vi "delete_Instrument.FrameworkTemplate.AppLauncher.vi"(8 "error in":errorcluster, 10 "Configuration Window? [T]":bool=TRUE, 11 "Debug Mode? [F]":bool) -> (0 "error out":errorcluster)   [LabVIEW 2019]
uses:
  <vilib>/JKI/JKI SMO/SMO/Typedefs/SMOState --Enum.ctl
  <userlib>/LevyLab/Instrument Framework/SMOs/Instrument/Instrument.lvclass
  C:/Program Files (x86)/National Instruments/LabVIEW 2019/vi.lib/JKI/JKI SMO/SMO/SMO.lvclass
  <userlib>/LevyLab/Instrument Framework/SMOs/Instrument UI/Instrument UI.lvclass
  C:/Program Files (x86)/National Instruments/LabVIEW 2019/vi.lib/JKI/JKI SMO/SMO.UI/SMO.UI.lvclass
  Instrument UI.FrameworkTemplate/Instrument UI.FrameworkTemplate.lvclass
  C:/Program Files (x86)/National Instruments/LabVIEW 2019/user.lib/LevyLab/Instrument Framework/SMOs/Instrument UI/Instrument UI.lvclass
  Instrument.FrameworkTemplate.lvclass
  C:/Program Files (x86)/National Instruments/LabVIEW 2019/user.lib/LevyLab/Instrument Framework/SMOs/Instrument/Instrument.lvclass
  <vilib>/JKI/JKI SMO/SMO/SMO.lvclass/SMO.ctl
  <vilib>/JKI/JKI SMO/SMO/Private/ReftoDVR--SMO.vi
  <vilib>/JKI/JKI SMO/SMO/SMO.lvclass
  <vilib>/JKI/JKI SMO/SMO.UI/SMO.UI.lvclass
panel:
  in  "Splash Status":string="Push Start to Start..." caption="String"
  in  "Start":bool=TRUE
  in  "Stop":bool=TRUE
  out "UI SMO State":T1=enum."Stopped"
  out "SMO State":T1
  # "Example Instrument SMO Test Launcher"
  # "For instructions on how to use the JKI State Machine Objects, examples and video tutorials, visit:\nhttp://jki.net/state-machine-objects/\n\nJKI State Machine Objects™\nhttp://jki.net/state-machine-objects/\nCopyright (C) 2005-2015, JKI <info@jki.net>\nALL RIGHTS RESERVED"
  # "Starting Example Instrument..."
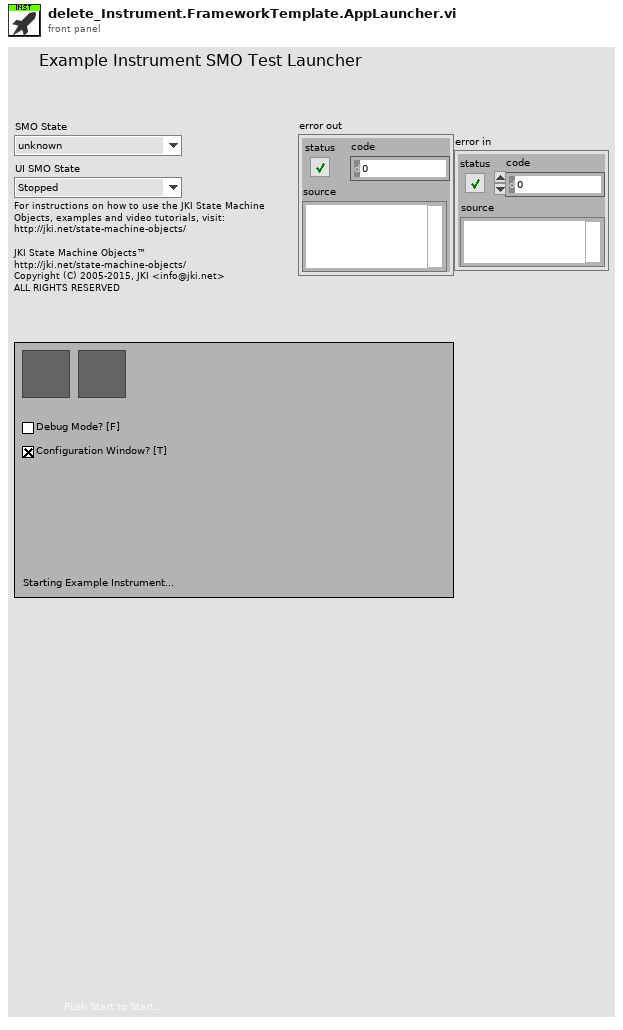
[diagram p1: front panel]
types:
  T1 = typedef "SMO.lvclass/SMOState --Enum.ctl" = enum16{"unknown", "Created", "Started", "Stopped"}
  T2 = enum32{"Invalid", "Standard", "Closed", "Hidden", "Minimized", "Maximized"}
  T3 = enum32{"invalid app kind", "Development System", "Run Time System", "Student Edition", "Embedded LabVIEW", "Evaluation", "Custom"}
  T4 = cluster{"Core":cluster{"Current VI Reference":refnum<vi>, "Close Panel on Exit?":bool}, "Instrument":refnum<class "Instrument.lvclass">, "Instrument UI":refnum<class "Instrument UI.lvclass">}
  T5 = cluster{"Current VI Reference":refnum<vi>, "Close Panel on Exit?":bool}
  T6 = typedef "SMO.lvclass/Public Events.ctl" = cluster{"Error":refnum<user-event>, "State":refnum<user-event>, "Reserve State":refnum<user-event>}
  T7 = cluster{"Event Registration Refnum":refnum<event-registration>, "Event Registration Refnum":refnum<event-registration>}
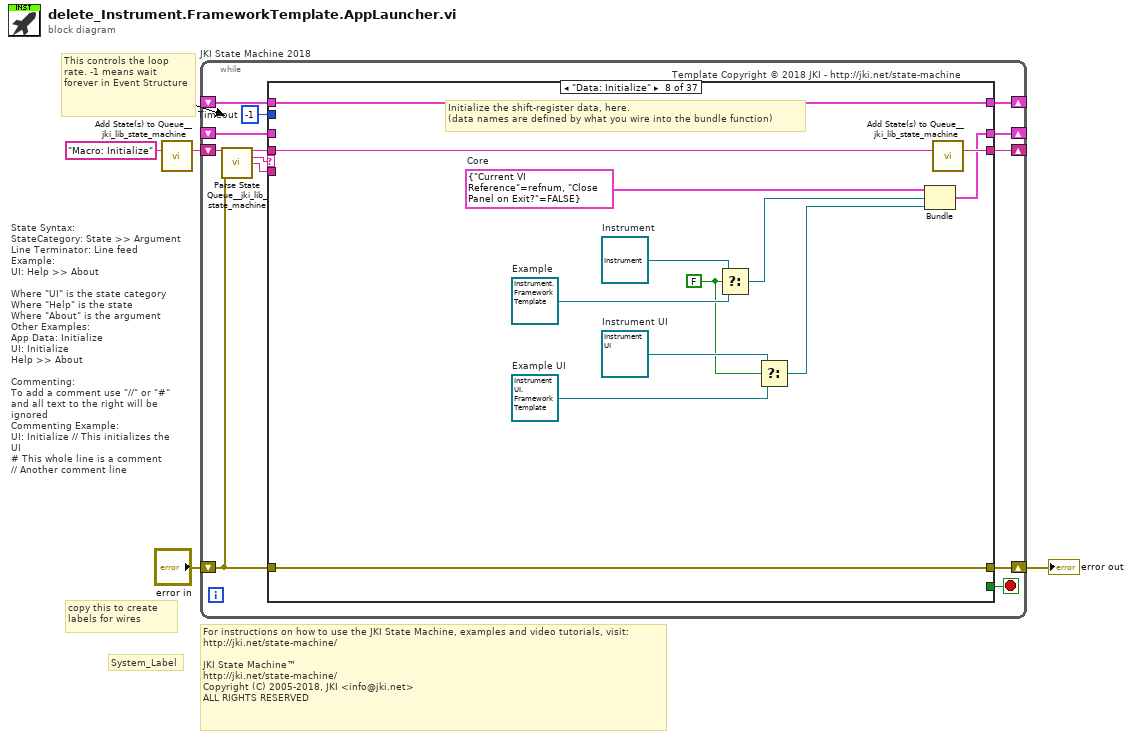
[diagram p0: block diagram]
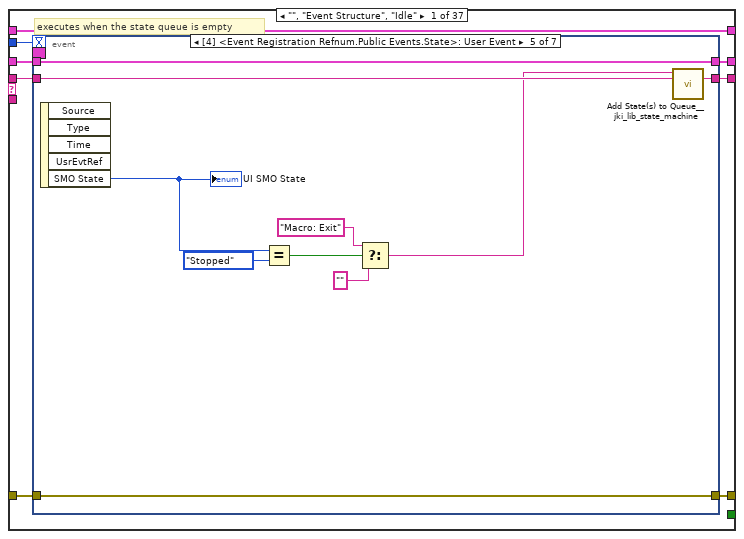
[diagram p2: hidden frame]
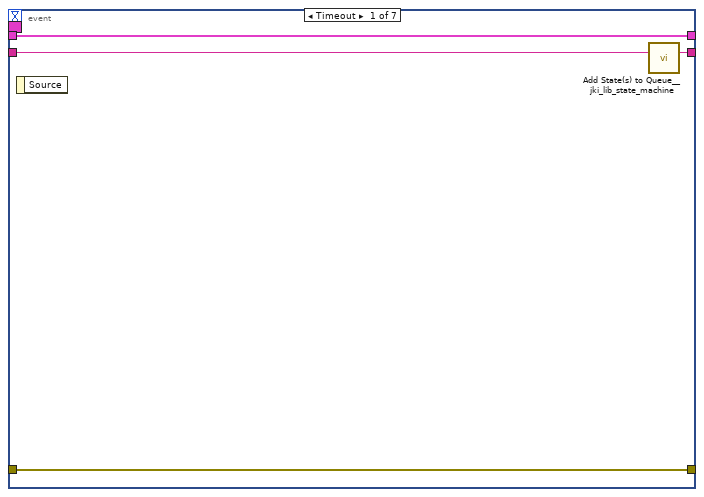
[diagram p3: hidden frame]
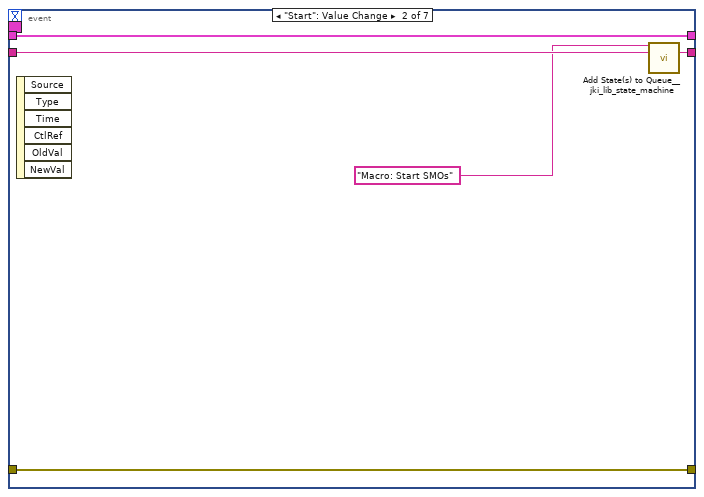
[diagram p4: hidden frame]
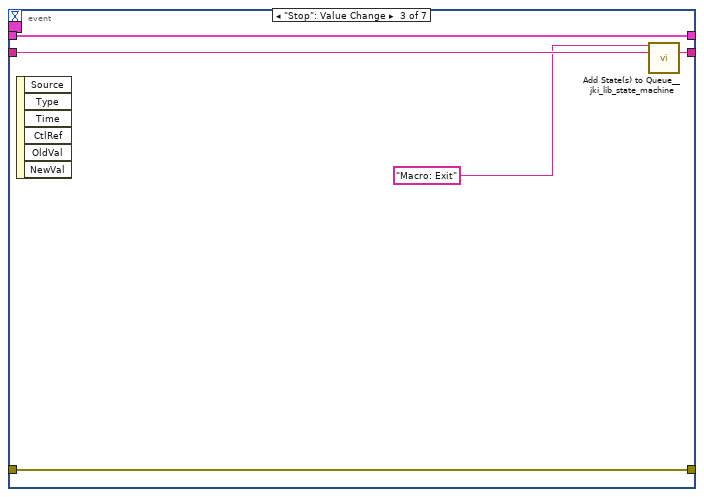
[diagram p5: hidden frame]
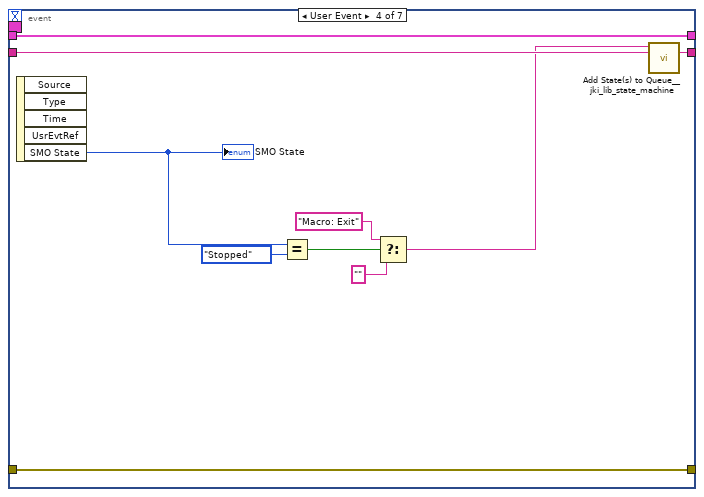
[diagram p6: hidden frame]
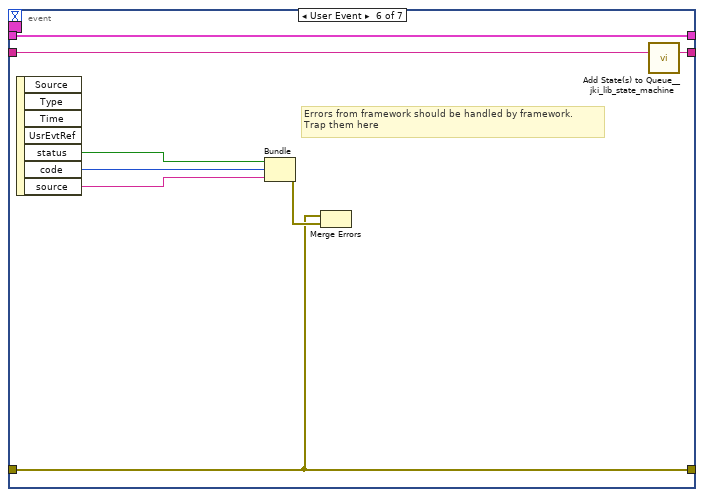
[diagram p7: hidden frame]
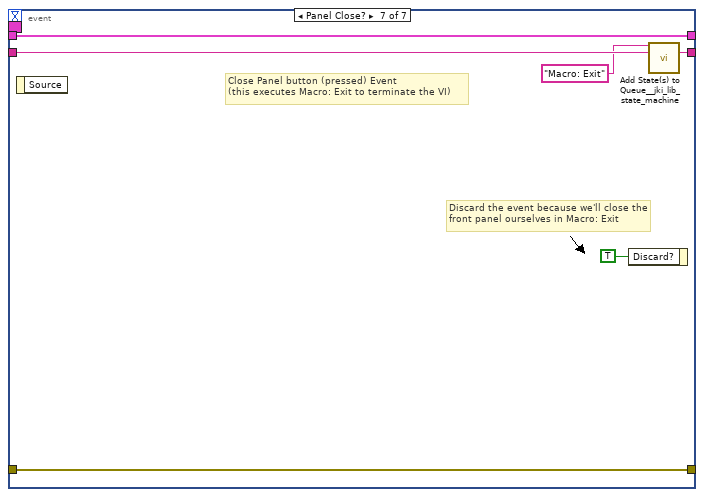
[diagram p8: hidden frame]
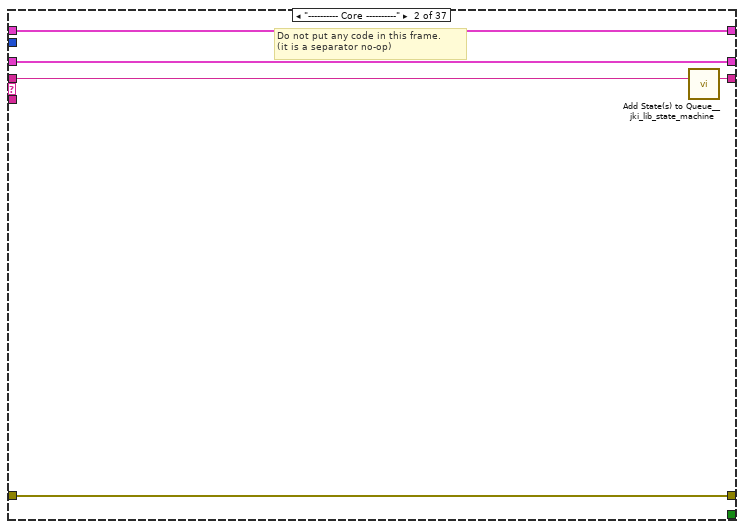
[diagram p9: hidden frame]
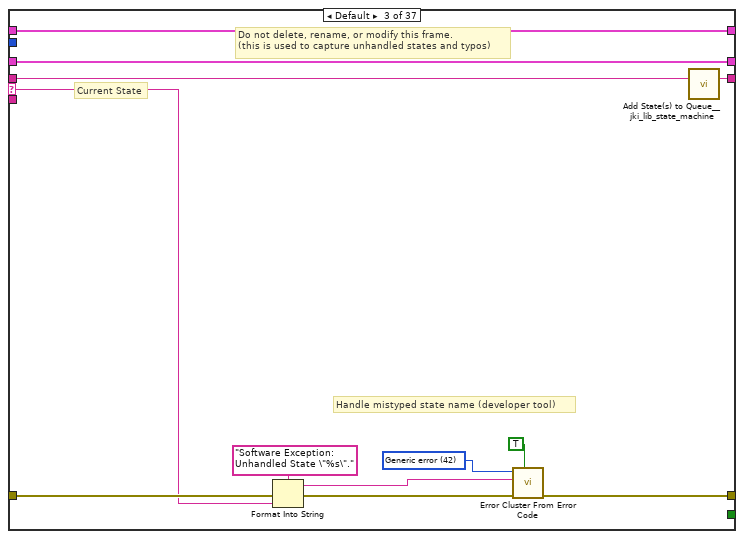
[diagram p10: hidden frame]
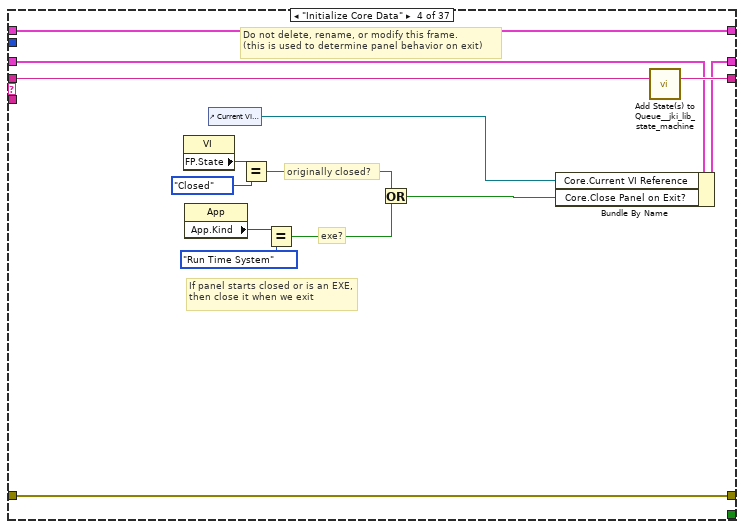
[diagram p11: hidden frame]
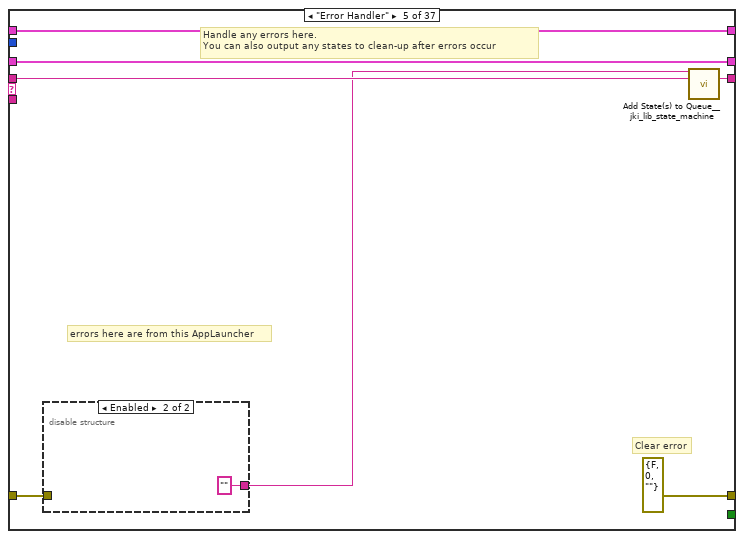
[diagram p12: hidden frame]
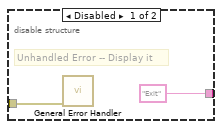
[diagram p13: hidden frame]
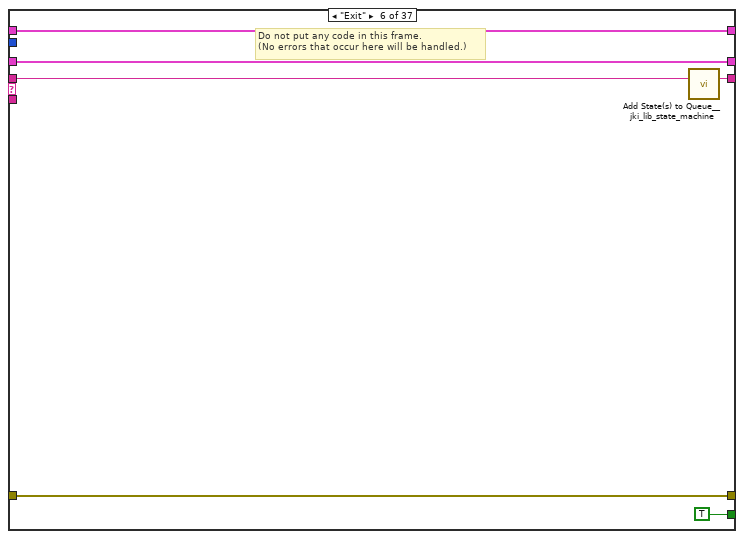
[diagram p14: hidden frame]
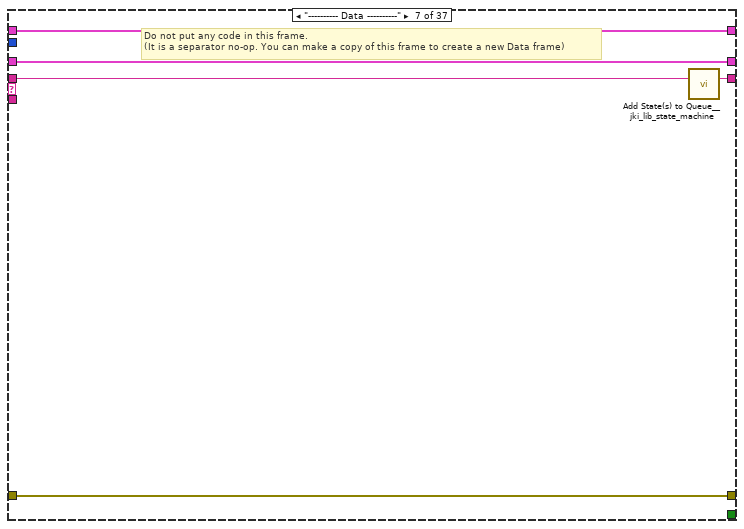
[diagram p15: hidden frame]
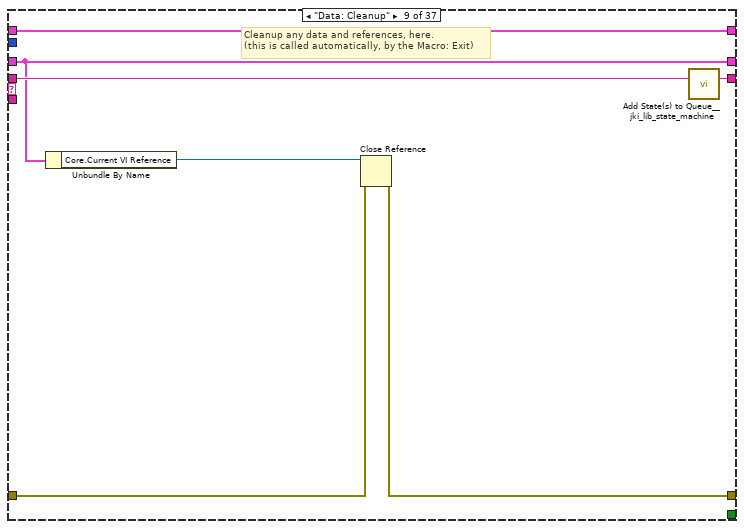
[diagram p16: hidden frame]
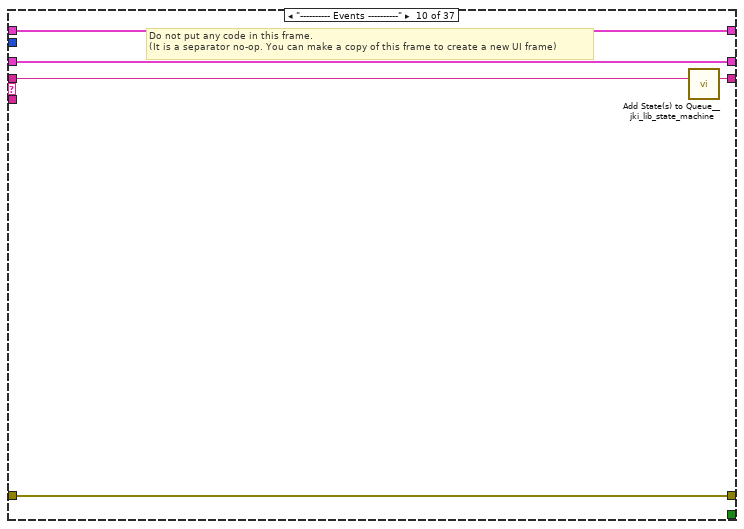
[diagram p17: hidden frame]
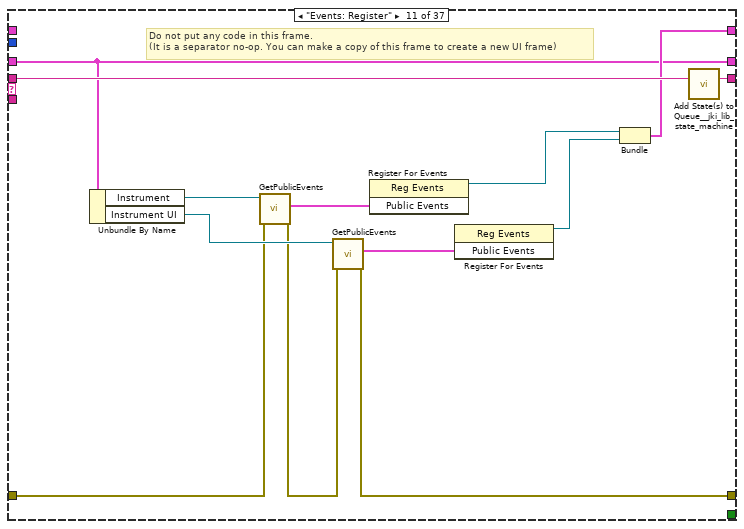
[diagram p18: hidden frame]
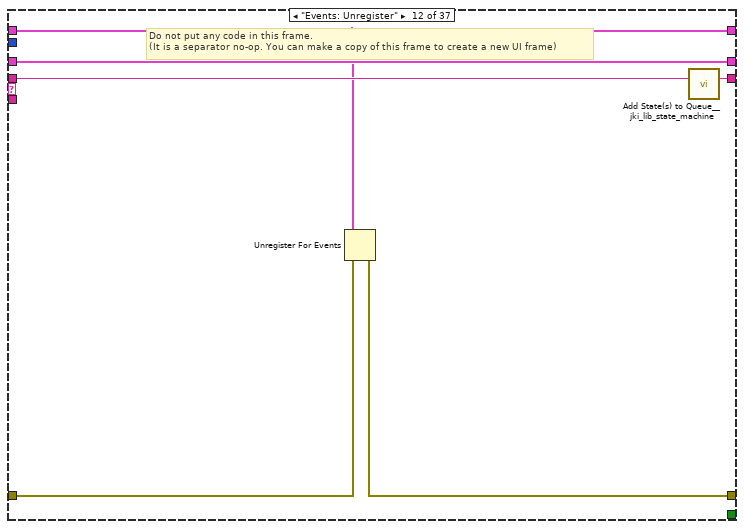
[diagram p19: hidden frame]
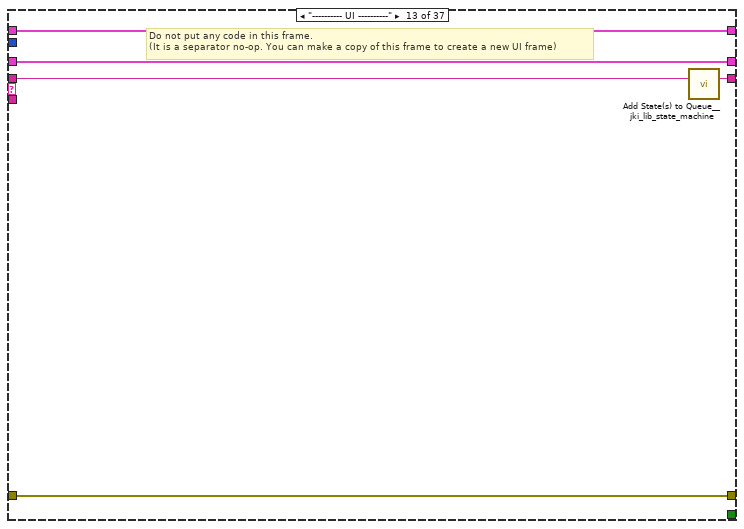
[diagram p20: hidden frame]
diagram:
  # "For instructions on how to use the JKI State Machine, examples and video tutorials, visit:\nhttp://jki.net/state-machine/\n\nJKI State Machine™\nhttp://jki.net/state-machine/\nCopyright (C) 2005-2018, JKI <info@jki.net>\nALL RIGHTS RESERVED"
  # "State Syntax:\nStateCategory: State >> Argument\nLine Terminator: Line feed\nExample:\nUI: Help >> About\n\nWhere \"UI\" is the state category\nWhere \"Help\" is the state\nWhere \"About\" is the argument\nOther Examples:\nApp Data: Initialize\nUI: Initialize\nHelp >> About\n\nCommenting:\nTo add a comment use \"//\" or \"#\" and all text to the right will be ignored\nCommenting Example:\nUI: Initialize // This initializes the UI\n# This whole line is a comment\n// Another comment line"
  # "copy this to create labels for wires"
  # "This controls the loop rate. -1 means wait forever in Event Structure"
  # "System_Label"
  n1 = call <vilib>:"Add State(s) to Queue__jki_lib_state_machine.vi"("State(s) in (\"\")"="Macro: Initialize") -> ("States Out"=w4:string)  [unwired: 14 in]
  n2 = while "JKI State Machine 2018" {
    shift-right: [w11] -> _
    shift-left: _ -> [w6]
    shift-right: [w14] -> w2
    shift-left: "error in" -> [w9]
    shift-right: [w13] -> _
    shift-left: w4 -> [w15]
    shift-right: [w8] -> _
    shift-left: _ -> [w7]
    stop <- w12 stop-if-true
    w10 = -1  # Timeout
    # "Template Copyright © 2018 JKI - http://jki.net/state-machine"
    n3 = call <vilib>:"Parse State Queue__jki_lib_state_machine.vi"("State Queue"=w15, "Error In (no error)"=w9) -> ("Remaining States"=w17:string, "Current State"=w5:string, "Arguments"=w16:string)  [unwired: 11 in]
    n4 = case shown="\"Data: Initialize\"" w5 {
      selector: w5 -> [_ _ w80 _ _ _ _ _ _ _ _ _ _ _ _ _ _ _ _ _ _ _ _ _ _ _ _ _ _ _ _ _ _ _ _ _ _]
      tunnel: w17 -> [w25 w78 w84 w104 w111 w120 w125 w138 w145 w150 w163 w169 w174 w180 w187 w199 w277 w282 w287 w293 w299 w305 w317 w322 w333 w342 w352 w359 w370 w385 w400 w415 w430 w445 w454 w461 w466]
      tunnel: w16 -> [_ _ _ _ _ _ _ _ _ _ _ _ _ _ w182 w193 _ _ _ _ _ _ _ _ _ _ _ _ _ _ _ _ _ _ _ w458 _]
      tunnel: [w22 w76 w86 w101 errorcluster {"status"=FALSE, "code"=0, "source"=""} ("error out") w117 w123 w133 w141 w148 w152 w164 w172 w175 w183 w196 w267 w280 w285 w291 w297 w303 w315 w320 w329 w334 w343 w353 w366 w381 w396 w412 w427 w442 w452 w456 w464] -> w14
      tunnel: w9 -> [w21 w76 w85 w101 w107 w117 w123 w133 w142 w148 w154 w165 w172 w177 w184 w197 w268 w280 w285 w291 w297 w303 w315 w320 w330 w335 w344 w354 w363 w377 w393 w410 w425 w438 w452 w457 w464]
      tunnel: [w24 w77 w83 w103 w110 w119 w124 w137 w144 w149 w162 w168 w173 w179 w186 w198 w276 w281 w286 w292 w298 w304 w316 w321 w332 w341 w351 w358 w369 w384 w399 w414 w429 w444 w453 w460 w465] -> w13
      tunnel: [_ _ _ _ _ TRUE _ _ _ _ _ _ _ _ _ _ _ _ _ _ _ _ _ _ _ _ _ _ _ _ _ _ _ _ _ _ _] -> w12
      tunnel: [w20 w75 w82 w102 w108 w118 w122 w136 w140 w147 w157 w167 w171 w178 w185 w195 w265 w279 w284 w290 w296 w302 w314 w319 w328 w337 w348 w356 w367 w382 w397 w411 w426 w441 w451 w459 w463] -> w11
      tunnel: w10 -> [w19 _ _ _ _ _ _ _ _ _ _ _ _ _ _ _ _ _ _ _ _ _ _ _ _ _ _ _ _ _ _ _ _ _ _ _ _]
      tunnel: [w18 w74 w79 w91 w106 w115 w121 w134 w139 w146 w160 w166 w170 w176 w181 w192 w266 w278 w283 w288 w295 w301 w308 w318 w331 w340 w350 w357 w368 w383 w398 w413 w428 w443 w450 w455 w462] -> w8
      tunnel: w7 -> [w18 w74 w79 w91 w106 w115 w121 w134 w139 w146 _ w166 w170 w176 w181 w192 w266 w278 w283 w288 w295 w301 w308 w318 w331 w340 w350 w357 w368 w383 w398 w413 w428 w443 w450 w455 w462]
      tunnel: w6 -> [w23 w75 w82 w97 w108 w118 w122 _ w140 w147 w157 w167 w171 w178 w185 w195 w265 w279 w284 w290 w296 w302 w314 w319 w326 w338 w349 w356 w367 w382 w397 w411 w426 w441 w451 w459 w463]
      frame "", "Event Structure", "Idle" {
        # "executes when the state queue is empty"
        n5 = event shown="[4] <Event Registration Refnum.Public Events.State>: User Event" {
          selector: w18 -> [_ _ _ _ _ _ _]
          dyn-events: _ -> [_ _ _ _ _ _ _]
          timeout: w19 -> [_ _ _ _ _ _ _]
          tunnel: w25 -> [w29 w34 w39 w49 w59 w67 w73]
          tunnel: [w28 w33 w38 w48 w58 w66 w72] -> w24
          tunnel: w23 -> [w26 w31 w36 w46 w56 w65 w70]
          tunnel: [w27 w32 w37 w47 w57 w60 w71] -> w22
          tunnel: w21 -> [w27 w32 w37 w47 w57 w60 w71]
          tunnel: [w26 w31 w36 w46 w56 w65 w70] -> w20
          event Timeout {
            n6 = event-data() -> ()  [unwired: 1 in, 1 out]
            n7 = call <vilib>:"Add State(s) to Queue__jki_lib_state_machine.vi"("State(s) in (\"\")"=w29) -> ("States Out"=w28:string)  [unwired: 14 in]
          }
          event "Start": Value Change {
            n8 = event-data() -> ()  [unwired: 1 in, 6 out]
            n9 = call <vilib>:"Add State(s) to Queue__jki_lib_state_machine.vi"("State(s) in Front (\"\")"="Macro: Start SMOs" ("State(s) in Front (\"\")"), "State(s) in (\"\")"=w34) -> ("States Out"=w33:string)  [unwired: 13 in]
          }
          event "Stop": Value Change {
            n10 = event-data() -> ()  [unwired: 1 in, 6 out]
            n11 = call <vilib>:"Add State(s) to Queue__jki_lib_state_machine.vi"("State(s) in Front (\"\")"="Macro: Exit" ("State(s) in Front (\"\")"), "State(s) in (\"\")"=w39) -> ("States Out"=w38:string)  [unwired: 13 in]
          }
          event User Event {
            n12 = event-data() -> ("SMO State"=w41:T1)  [unwired: 1 in, 4 out]
            "SMO State" <- w41
            n13 = Equal?(x=w41, y=SMOState_--Enum."Stopped") -> (x = y?=w44:bool)
            n14 = Select(t="Macro: Exit", s=w44, f="" ("State(s) in Front (\"\")")) -> (s? t:f=w40:string)
            n15 = call <vilib>:"Add State(s) to Queue__jki_lib_state_machine.vi"("State(s) in Front (\"\")"=w40, "State(s) in (\"\")"=w49) -> ("States Out"=w48:string)  [unwired: 13 in]
          }
          event User Event {
            n16 = event-data() -> ("SMO State"=w50:T1)  [unwired: 1 in, 4 out]
            "UI SMO State" <- w50
            n17 = Equal?(x=w50, y=SMOState_--Enum."Stopped") -> (x = y?=w54:bool)
            n18 = Select(t="Macro: Exit", s=w54, f="" ("State(s) in Front (\"\")")) -> (s? t:f=w52:string)
            n19 = call <vilib>:"Add State(s) to Queue__jki_lib_state_machine.vi"("State(s) in Front (\"\")"=w52, "State(s) in (\"\")"=w59) -> ("States Out"=w58:string)  [unwired: 13 in]
          }
          event User Event {
            # "Errors from framework should be handled by framework.\nTrap them here"
            n20 = event-data() -> ("status"=w61:bool, "code"=w63:i32, "source"=w62:string)  [unwired: 1 in, 4 out]
            n21 = Bundle("status"=w61, "code"=w63, "source"=w62) -> (w64:errorcluster)  [unwired: 1 in]
            n22 = Merge Errors(w60, w64) -> ()  [unwired: 1 out]
            n23 = call <vilib>:"Add State(s) to Queue__jki_lib_state_machine.vi"("State(s) in (\"\")"=w67) -> ("States Out"=w66:string)  [unwired: 14 in]
          }
          event Panel Close? {
            # "Discard the event because we'll close the front panel ourselves in Macro: Exit"
            # "Close Panel button (pressed) Event\n(this executes Macro: Exit to terminate the VI)"
            n24 = event-data() -> ()  [unwired: 1 in, 1 out]
            n25 = event-data("Discard?"=TRUE) -> ()  [unwired: 1 in, 1 out]
            n26 = call <vilib>:"Add State(s) to Queue__jki_lib_state_machine.vi"("State(s) in Front (\"\")"="Macro: Exit", "State(s) in (\"\")"=w73) -> ("States Out"=w72:string)  [unwired: 13 in]
          }
        }
      }
      frame "---------- Core ----------" {
        # "Do not put any code in this frame.\n(it is a separator no-op)"
        n27 = call <vilib>:"Add State(s) to Queue__jki_lib_state_machine.vi"("State(s) in (\"\")"=w78) -> ("States Out"=w77:string)  [unwired: 14 in]
      }
      frame Default {
        w89 = 42 items=["No error", "Argument error", "Memory is full", "Out of zone", "End of file", "File already open", "Generic file I/O error", "File not found", "File permission error", "Disk is full", "Duplicate path", "Too many files open", "System feature not enabled", "Resource file not found", "Cannot add resource", "Resource not found", "Image not found", "Image memory error", "Pen does not exist", "Config type invalid", "Config token not found", "Config parse error", "Config memory error", "Bad external code format", "Bad external code offset", "External code not present", "Null window", "Destroy window error", "Null menu", "Print aborted", "Bad print record", "Print driver error", "Windows error during printing", "Memory error during printing", "Print dialog error", "Generic print error", "Invalid device refnum", "Device not found", "Device parameter error", "Device unit error", "Cannot open device", "Device call aborted", "Generic error", "Cancelled by user", "Object ID too low", "Object ID too high", "Object not in heap", "Unknown heap", "Unknown object (invalid DefProc)", "Unknown object (DefProc not in table)", "Message out of range", "Invalid (null) method", "Unknown message", "Manager call not supported", "Bad address", "Network operation in progress", "Network operation timed out", "Connection is busy", "Network attribute not supported", "Network error", "Address in use", "System out of memory", "Connection aborted", "Connection refused", "Not connected", "Already connected", "Connection closed", "Initialization error (interapplication manager)", "Bad occurrence", "Wait on unbound occurrence handler", "Occurrence queue overflow", "Datalog type conflict", "Unused", "Unrecognized type (interapplication manager)", "Memory corrupt", "Failed to make temporary DLL", "Old CIN version", "Drag socket not found", "Failed to load drop-object", "Failed to register OLE object", "Failed to release OLE object", "Format specifier type mismatch", "Unknown format specifier", "Too few format specifiers", "Too many format specifiers", "Scan failed", "Newer CIN version", "Error converting to variant", "Runtime menu error", "Password tampered", "Variant attribute not found", "Incompatible variant data type", "Event data is not available", "Event Store is not present", "Occurrence is not found", "Event Queue is not created", "Event info is not available", "Refnum passed is NULL", "Error retrieving Class GUID", "Error retrieving CoClass GUID", "Error retrieving TypeLib GUID.", "Bad built application magic bytes.", "Specific driver is different from the specific driver associated with the Logical Name.", "There is no session opened to the class driver.", "Max Error", "MAX - Error with config objects", "MAX - Error loading configuration", "MAX - Group not supported"]
        # "Current State"
        # "Do not delete, rename, or modify this frame.\n(this is used to capture unhandled states and typos)"
        # "Handle mistyped state name (developer tool)"
        n28 = Format Into String(format string="Software Exception: Unhandled State \"%s\"." ("message"), error in=w85, w80) -> (resulting string=w88:string, error out=w87:errorcluster)  [unwired: 1 in]
        n29 = call <vilib>:"Error Cluster From Error Code.vi"("show call chain? (False)"=TRUE, "error in (no error)"=w87, "error message (\"\")"=w88, "error code (0)"=w89) -> ("error out"=w86:errorcluster)  [unwired: 5 in]
        n30 = call <vilib>:"Add State(s) to Queue__jki_lib_state_machine.vi"("State(s) in (\"\")"=w84) -> ("States Out"=w83:string)  [unwired: 14 in]
      }
      frame "Initialize Core Data" {
        # "Do not delete, rename, or modify this frame.\n(this is used to determine panel behavior on exit)"
        # "originally closed?"
        # "exe?"
        # "If panel starts closed or is an EXE, then close it when we exit"
        n31 = property class="VI"() -> ("FP.State"=w94:T2)  [unwired: 2 in, 2 out]
        n32 = property class="App"() -> ("App.Kind"=w100:T3)  [unwired: 2 in, 2 out]
        n33 = control-ref of="Current VI Reference"() -> (w95:refnum<vi>)
        n34 = Equal?(x=w94, y=T2."Closed" ("Front Panel Window:State")) -> (x = y?=w92:bool)
        n35 = Equal?(x=w100, y=T3."Run Time System" ("Application:Kind")) -> (x = y?=w98:bool)
        n36 = Or(x=w92, y=w98) -> (x .or. y?=w96:bool)
        n37 = Bundle By Name(cluster=w97, "Core.Current VI Reference"=w95, "Core.Close Panel on Exit?"=w96) -> (w102:T4)
        n38 = call <vilib>:"Add State(s) to Queue__jki_lib_state_machine.vi"("State(s) in (\"\")"=w104) -> ("States Out"=w103:string)  [unwired: 14 in]
      }
      frame "Error Handler" {
        # "errors here are from this AppLauncher"
        # "Handle any errors here.\nYou can also output any states to clean-up after errors occur"
        # "Clear error"
        n39 = disable-structure shown="Enabled" {
          disable-tunnel: w107 -> [w113 _]
          disable-tunnel: ["Exit" "" ("State(s) in Front (\"\")")] -> w105
          frame Disabled {
            # "Unhandled Error -- Display it"
            n40 = call <vilib>:"General Error Handler.vi"("error in (no error)"=w113) -> ()  [unwired: 10 in, 5 out]
          }
          frame Enabled {
          }
        }
        n41 = call <vilib>:"Add State(s) to Queue__jki_lib_state_machine.vi"("State(s) in Front (\"\")"=w105, "State(s) in (\"\")"=w111) -> ("States Out"=w110:string)  [unwired: 13 in]
      }
      frame "Exit" {
        # "Do not put any code in this frame.\n(No errors that occur here will be handled.)"
        n42 = call <vilib>:"Add State(s) to Queue__jki_lib_state_machine.vi"("State(s) in (\"\")"=w120) -> ("States Out"=w119:string)  [unwired: 14 in]
      }
      frame "---------- Data ----------" {
        # "Do not put any code in this frame.\n(It is a separator no-op. You can make a copy of this frame to create a new Data frame)"
        n43 = call <vilib>:"Add State(s) to Queue__jki_lib_state_machine.vi"("State(s) in (\"\")"=w125) -> ("States Out"=w124:string)  [unwired: 14 in]
      }
      frame "Data: Initialize" {
        w126 = FALSE ("s")
        w129 = refnum<class "Instrument.FrameworkTemplate.lvclass"> refnum  # Example
        w130 = refnum<class "Instrument UI.FrameworkTemplate.lvclass"> refnum  # Example UI
        w131 = refnum<class "Instrument UI.lvclass"> refnum  # Instrument UI
        w132 = refnum<class "Instrument.lvclass"> refnum  # Instrument
        w135 = T5 {"Current VI Reference"=refnum, "Close Panel on Exit?"=FALSE}  # Core
        # "Initialize the shift-register data, here.\n(data names are defined by what you wire into the bundle function)"
        n44 = Select(t=w132, s=w126, f=w129) -> (s? t:f=w128:refnum<class "Instrument.lvclass">)
        n45 = Select(t=w131, s=w126, f=w130) -> (s? t:f=w127:refnum<class "Instrument UI.lvclass">)
        n46 = Bundle("Core"=w135, "Instrument"=w128, "Instrument UI"=w127) -> (w136:T4)  [unwired: 1 in]
        n47 = call <vilib>:"Add State(s) to Queue__jki_lib_state_machine.vi"("State(s) in (\"\")"=w138) -> ("States Out"=w137:string)  [unwired: 14 in]
      }
      frame "Data: Cleanup" {
        # "Cleanup any data and references, here.\n(this is called automatically, by the Macro: Exit)"
        n48 = Unbundle By Name(w140) -> ("Core.Current VI Reference"=w143:refnum<vi>)
        n49 = Close Reference(reference=w143, error in (no error)=w142) -> (error out=w141:errorcluster)
        n50 = call <vilib>:"Add State(s) to Queue__jki_lib_state_machine.vi"("State(s) in (\"\")"=w145) -> ("States Out"=w144:string)  [unwired: 14 in]
      }
      frame "---------- Events ----------" {
        # "Do not put any code in this frame.\n(It is a separator no-op. You can make a copy of this frame to create a new UI frame)"
        n51 = call <vilib>:"Add State(s) to Queue__jki_lib_state_machine.vi"("State(s) in (\"\")"=w150) -> ("States Out"=w149:string)  [unwired: 14 in]
      }
      frame "Events: Register" {
        # "Do not put any code in this frame.\n(It is a separator no-op. You can make a copy of this frame to create a new UI frame)"
        n52 = Unbundle By Name(w157) -> ("Instrument"=w156:refnum<class "Instrument.lvclass">, "Instrument UI"=w155:refnum<class "Instrument UI.lvclass">)
        n53 = call <vilib>:"GetPublicEvents.vi"("error in (no error)"=w154, "SMO"=w156) -> ("error out"=w153:errorcluster, "Public Events"=w158:T6)  [unwired: 7 in, 1 out]
        n54 = call <vilib>:"GetPublicEvents.vi"("error in (no error)"=w153, "SMO"=w155) -> ("error out"=w152:errorcluster, "Public Events"=w159:T6)  [unwired: 7 in, 1 out]
        n55 = register-events(w158) -> (reference out=w161:refnum<event-registration>)  [unwired: 2 in, 1 out]
        n56 = register-events(w159) -> (reference out=w151:refnum<event-registration>)  [unwired: 2 in, 1 out]
        n57 = Bundle("Event Registration Refnum"=w161, "Event Registration Refnum"=w151) -> (w160:T7)  [unwired: 1 in]
        n58 = call <vilib>:"Add State(s) to Queue__jki_lib_state_machine.vi"("State(s) in (\"\")"=w163) -> ("States Out"=w162:string)  [unwired: 14 in]
      }
      frame "Events: Unregister" {
        # "Do not put any code in this frame.\n(It is a separator no-op. You can make a copy of this frame to create a new UI frame)"
        n59 = Unregister For Events(event registration refnum=w166, error in=w165) -> (error out=w164:errorcluster)
        n60 = call <vilib>:"Add State(s) to Queue__jki_lib_state_machine.vi"("State(s) in (\"\")"=w169) -> ("States Out"=w168:string)  [unwired: 14 in]
      }
      frame "---------- UI ----------" {
        # "Do not put any code in this frame.\n(It is a separator no-op. You can make a copy of this frame to create a new UI frame)"
        n61 = call <vilib>:"Add State(s) to Queue__jki_lib_state_machine.vi"("State(s) in (\"\")"=w174) -> ("States Out"=w173:string)  [unwired: 14 in]
      }
      frame "UI: Initialize" {
        # "Initialize the User Interface, here.\n(this is called automatically, by the Macro: Init)"
        n62 = invoke on="Stop" class="Bool (strict)" method="Reinit To Default"() -> ()  [unwired: 3 in, 3 out]
        n63 = invoke on="error out" class="Clust (strict)" method="Reinit To Default"() -> ()  [unwired: 3 in, 3 out]
        n64 = invoke on="SMO State 2" class="Enum (strict)" method="Reinit To Default"() -> ()  [unwired: 3 in, 3 out]
        n65 = invoke on="Start" class="Bool (strict)" method="Reinit To Default"() -> ()  [unwired: 3 in, 3 out]
        n66 = call <userlib>:"Fit VI window to Largest Dec__ogtk.vi"("error in (no error)"=w177) -> ("error out"=w175:errorcluster)  [unwired: 5 in, 1 out]
        n67 = call <vilib>:"Add State(s) to Queue__jki_lib_state_machine.vi"("State(s) in (\"\")"=w180) -> ("States Out"=w179:string)  [unwired: 14 in]
      }
      frame "UI: Cursor Set" {
        # "Argument"
        # "Set and Unset Cursor Busy.\n(Usage: \"UI: Cursor Set >> Busy|Idle\")"
        n68 = case shown="\"Busy\"" w182 {
          tunnel: w184 -> [w189 w191]
          tunnel: [w188 w190] -> w183
          frame "Idle", Default {
            n69 = call <vilib>:"Unset Busy.vi"("error in (no error)"=w189) -> ("error out"=w188:errorcluster)  [unwired: 10 in]
          }
          frame "Busy" {
            n70 = call <vilib>:"Set Busy.vi"("error in (no error)"=w191) -> ("error out"=w190:errorcluster)  [unwired: 9 in, 1 out]
          }
        }
        n71 = call <vilib>:"Add State(s) to Queue__jki_lib_state_machine.vi"("State(s) in (\"\")"=w187) -> ("States Out"=w186:string)  [unwired: 14 in]
      }
      frame "UI: Front Panel State" {
        # "Argument"
        # "Set Front Panel Open or Closed\n(Usage: \"UI: Front Panel State >> Open|Close\")"
        n72 = Unbundle By Name(w195) -> ("Core.Current VI Reference"=w194:refnum<vi>)
        n73 = case shown="\"Open\", \"Standard\", Default" w193 {
          tunnel: w197 -> [w205 w220 w231 w244 w257]
          tunnel: [w207 w221 w233 w246 w259] -> w196
          tunnel: w194 -> [w206 w218 w232 w245 w258]
          frame "Open", "Standard", Default {
            w200 = T2."Standard" ("State")
            n74 = property class="VI"(reference=w206, error in=w205) -> (reference out=w203:refnum<vi>, error out=w204:errorcluster, "FP.State"=w202:T2)
            n75 = Not Equal?(x=w202, y=w200) -> (x != y?=w201:bool)
            n76 = case shown="False" w201 {
              tunnel: [w211 w213] -> w207
              tunnel: w204 -> [w210 w213]
              tunnel: w203 -> [w209 _]
              tunnel: w200 -> [w208 _]
              frame True {
                n77 = invoke class="VI" method="FP.Open"(reference=w209, error in=w210, "Activate"=TRUE, "State"=w208) -> (error out=w211:errorcluster)  [unwired: 1 in, 4 out]
              }
              frame False {
              }
            }
          }
          frame "Close", "Closed" {
            n78 = property class="VI"(reference=w218, error in=w220) -> (reference out=w217:refnum<vi>, error out=w219:errorcluster, "FP.State"=w215:T2)
            n79 = Not Equal?(x=w215, y=T2."Closed" ("Front Panel Window:State")) -> (x != y?=w214:bool)
            n80 = case shown="True" w214 {
              tunnel: [w222 w225] -> w221
              tunnel: w219 -> [w222 w224]
              tunnel: w217 -> [_ w223]
              frame False {
              }
              frame True {
                n81 = invoke class="VI" method="FP.Close"(reference=w223, error in=w224) -> (error out=w225:errorcluster)  [unwired: 1 in, 2 out]
              }
            }
          }
          frame "Hidden", "Hide" {
            w226 = T2."Hidden" ("State")
            n82 = property class="VI"(reference=w232, error in=w231) -> (reference out=w229:refnum<vi>, error out=w230:errorcluster, "FP.State"=w228:T2)
            n83 = Not Equal?(x=w228, y=w226) -> (x != y?=w227:bool)
            n84 = case shown="True" w227 {
              tunnel: [w237 w238] -> w233
              tunnel: w230 -> [w236 w238]
              tunnel: w229 -> [w235 _]
              tunnel: w226 -> [w234 _]
              frame True {
                n85 = invoke class="VI" method="FP.Open"(reference=w235, error in=w236, "State"=w234) -> (error out=w237:errorcluster)  [unwired: 2 in, 4 out]
              }
              frame False {
              }
            }
          }
          frame "Minimize", "Minimized" {
            w239 = T2."Minimized" ("State")
            n86 = property class="VI"(reference=w245, error in=w244) -> (reference out=w242:refnum<vi>, error out=w243:errorcluster, "FP.State"=w241:T2)
            n87 = Not Equal?(x=w241, y=w239) -> (x != y?=w240:bool)
            n88 = case shown="True" w240 {
              tunnel: [w250 w251] -> w246
              tunnel: w243 -> [w249 w251]
              tunnel: w242 -> [w248 _]
              tunnel: w239 -> [w247 _]
              frame True {
                n89 = invoke class="VI" method="FP.Open"(reference=w248, error in=w249, "State"=w247) -> (error out=w250:errorcluster)  [unwired: 2 in, 4 out]
              }
              frame False {
              }
            }
          }
          frame "Maximize", "Maximized" {
            w252 = T2."Maximized" ("State")
            n90 = property class="VI"(reference=w258, error in=w257) -> (reference out=w255:refnum<vi>, error out=w256:errorcluster, "FP.State"=w254:T2)
            n91 = Not Equal?(x=w254, y=w252) -> (x != y?=w253:bool)
            n92 = case shown="True" w253 {
              tunnel: [w263 w264] -> w259
              tunnel: w256 -> [w262 w264]
              tunnel: w255 -> [w261 _]
              tunnel: w252 -> [w260 _]
              frame True {
                n93 = invoke class="VI" method="FP.Open"(reference=w261, error in=w262, "State"=w260) -> (error out=w263:errorcluster)  [unwired: 2 in, 4 out]
              }
              frame False {
              }
            }
          }
        }
        n94 = call <vilib>:"Add State(s) to Queue__jki_lib_state_machine.vi"("State(s) in (\"\")"=w199) -> ("States Out"=w198:string)  [unwired: 14 in]
      }
      frame "UI: Set Background Color" {
        # "Do not put any code in this frame.\n(It is a separator no-op. You can make a copy of this frame to create a new UI frame)"
        n95 = property class="VI"(error in=w268) -> (error out=w270:errorcluster, "Panel"=w271:refnum<vi>)  [unwired: 1 in, 1 out]
        n96 = property class="Pnl"(reference=w271, error in=w270) -> (error out=w269:errorcluster, "Panes[]"=w272:refnum<vi>[])  [unwired: 1 out]
        n97 = Index Array(array=w272, index=0) -> (element=w274:refnum<vi>)
        n98 = property class="Pane"(reference=w274, error in=w269, "PaneColor"=u32 16777238 ("Color Box")) -> (error out=w267:errorcluster)  [unwired: 1 out]
        n99 = call <vilib>:"Add State(s) to Queue__jki_lib_state_machine.vi"("State(s) in (\"\")"=w277) -> ("States Out"=w276:string)  [unwired: 14 in]
      }
      frame "UI: Exit" {
        # "Do not put any code in this frame.\n(It is a separator no-op. You can make a copy of this frame to create a new UI frame)"
        n100 = invoke on="Start" class="Bool (strict)" method="Reinit To Default"() -> ()  [unwired: 3 in, 3 out]
        n101 = invoke on="Stop" class="Bool (strict)" method="Reinit To Default"() -> ()  [unwired: 3 in, 3 out]
        n102 = call <vilib>:"Add State(s) to Queue__jki_lib_state_machine.vi"("State(s) in (\"\")"=w282) -> ("States Out"=w281:string)  [unwired: 14 in]
      }
      frame "---------- Macro ----------" {
        # "Do not put any code in this frame.\n(It is a separator no-op. You can make a copy of this frame to create a new Macro frame)"
        n103 = call <vilib>:"Add State(s) to Queue__jki_lib_state_machine.vi"("State(s) in (\"\")"=w287) -> ("States Out"=w286:string)  [unwired: 14 in]
      }
      frame "Macro: Initialize" {
        # "Initialization Macro\n(This is called once, when the VI starts)"
        n104 = call <vilib>:"Add State(s) to Queue__jki_lib_state_machine.vi"("State(s) in Front (\"\")"="Data: Initialize\nInitialize Core Data\n//Events: Register\nUI: Initialize\nUI: Front Panel State >> Open\nUI: Set Background Color\nSplash: Set Status >> Push Start to Start...", "State(s) in (\"\")"=w293) -> ("States Out"=w292:string)  [unwired: 13 in]
      }
      frame "Macro: Start SMOs" {
        # "Do not put any code in this frame.\n(It is a separator no-op. You can make a copy of this frame to create a new Macro frame)"
        n105 = call <vilib>:"Add State(s) to Queue__jki_lib_state_machine.vi"("State(s) in Front (\"\")"="Splash: Set Status >> Starting Instrument...\nSMO: Create Instrument\nSMO: Create Instrument UI\nEvents: Register\nSMO: Start Instrument\nSplash: Set Status >> Instrument Process Started...\nSplash: Set Status >> Starting User Interface...\nSMO: Start Instrument UI\nUI: Front Panel State >> Hide\nSMO: Show Instrument UI" ("State(s) in Front (\"\")"), "State(s) in (\"\")"=w299) -> ("States Out"=w298:string)  [unwired: 13 in]
      }
      frame "Macro: Stop SMOs" {
        # "Do not put any code in this frame.\n(It is a separator no-op. You can make a copy of this frame to create a new Macro frame)"
        n106 = call <vilib>:"Add State(s) to Queue__jki_lib_state_machine.vi"("State(s) in Front (\"\")"="SMO: Stop Instrument\nSMO: Destroy Instrument\nSMO: Hide Instrument UI\nSMO: Stop Instrument UI\nSMO: Destroy Instrument UI" ("State(s) in Front (\"\")"), "State(s) in (\"\")"=w305) -> ("States Out"=w304:string)  [unwired: 13 in]
      }
      frame "Macro: Exit" {
        # "Exit Macro\n(This is called once, when the VI exits)"
        n107 = Unbundle By Name(w314) -> ("Core.Close Panel on Exit?"=w313:bool)
        n108 = Select(t="UI: Front Panel State >> Open", s=w313, f="") -> (s? t:f=w310:string)
        n109 = call <vilib>:"Add State(s) to Queue__jki_lib_state_machine.vi"("State(s) in Front (\"\")"="UI: Front Panel State >> Open\nUI: Exit", "State(s) in (\"\")"=w310, "State(s) at Back (\"\")"="Macro: Stop SMOs\nData: Cleanup\nEvents: Unregister\nExit") -> ("States Out"=w309:string)  [unwired: 12 in]
        n110 = call <vilib>:"Add State(s) to Queue__jki_lib_state_machine.vi"("State(s) in Front (\"\")"=w309, "State(s) in (\"\")"=w317) -> ("States Out"=w316:string)  [unwired: 13 in]
      }
      frame "---------- SMO ----------" {
        # "Do not put any code in this frame.\n(It is a separator no-op. You can make a copy of this frame to create a new Macro frame)"
        n111 = call <vilib>:"Add State(s) to Queue__jki_lib_state_machine.vi"("State(s) in (\"\")"=w322) -> ("States Out"=w321:string)  [unwired: 14 in]
      }
      frame "SMO: Create Instrument" {
        # "Do not put any code in this frame.\n(It is a separator no-op. You can make a copy of this frame to create a new Macro frame)"
        n112 = Unbundle By Name(w326) -> ("Instrument"=w325:refnum<class "Instrument.lvclass">)
        n113 = call-dynamic "Create Instrument SMO.vi"("error in (no error)"=w330, "Debug Mode? [F]"="Debug Mode? [F]", "Configuration Window? [T]"="Configuration Window? [T]", "Instrument in"=w325) -> ("error out"=w329:errorcluster, "Instrument out"=w327:refnum<class "Instrument.lvclass">)  [unwired: 6 in]
        n114 = Bundle By Name(cluster=w326, "Instrument"=w327) -> (w328:T4)
        n115 = call <vilib>:"Add State(s) to Queue__jki_lib_state_machine.vi"("State(s) in (\"\")"=w333) -> ("States Out"=w332:string)  [unwired: 14 in]
      }
      frame "SMO: Start Instrument" {
        # "Do not put any code in this frame.\n(It is a separator no-op. You can make a copy of this frame to create a new Macro frame)"
        n116 = Unbundle By Name(w338) -> ("Instrument"=w339:refnum<class "Instrument.lvclass">)
        n117 = call <vilib>:"Start.vi"("error in (no error)"=w335, "SMO"=w339) -> ("error out"=w334:errorcluster, "SMO out"=w336:refnum<class "Instrument.lvclass">)  [unwired: 8 in]
        n118 = Bundle By Name(cluster=w338, "Instrument"=w336) -> (w337:T4)
        n119 = call <vilib>:"Add State(s) to Queue__jki_lib_state_machine.vi"("State(s) in (\"\")"=w342) -> ("States Out"=w341:string)  [unwired: 14 in]
      }
      frame "SMO: Create Instrument UI" {
        # "Do not put any code in this frame.\n(It is a separator no-op. You can make a copy of this frame to create a new Macro frame)"
        n120 = Unbundle By Name(w349) -> ("Instrument UI"=w347:refnum<class "Instrument UI.lvclass">, "Instrument"=w346:refnum<class "Instrument.lvclass">)
        n121 = call <userlib>:"Create UI.vi"("error in (no error)"=w344, "Instrument in"=w346, "Instrument UI"=w347) -> ("error out"=w343:errorcluster, "Instrument UI out"=w345:refnum<class "Instrument UI.lvclass">)  [unwired: 7 in]
        n122 = Bundle By Name(cluster=w349, "Instrument UI"=w345) -> (w348:T4)
        n123 = call <vilib>:"Add State(s) to Queue__jki_lib_state_machine.vi"("State(s) in (\"\")"=w352) -> ("States Out"=w351:string)  [unwired: 14 in]
      }
      frame "SMO: Start Instrument UI" {
        # "Do not put any code in this frame.\n(It is a separator no-op. You can make a copy of this frame to create a new Macro frame)"
        n124 = Unbundle By Name(w356) -> ("Instrument UI"=w355:refnum<class "Instrument UI.lvclass">)
        n125 = call <vilib>:"Start.vi"("error in (no error)"=w354, "SMO"=w355) -> ("error out"=w353:errorcluster)  [unwired: 8 in, 1 out]
        n126 = call <vilib>:"Add State(s) to Queue__jki_lib_state_machine.vi"("State(s) in (\"\")"=w359) -> ("States Out"=w358:string)  [unwired: 14 in]
      }
      frame "SMO: Show Instrument UI" {
        # "Do not put any code in this frame.\n(It is a separator no-op. You can make a copy of this frame to create a new Macro frame)"
        n127 = Unbundle By Name(w367) -> ("Instrument UI"=w365:refnum<class "Instrument UI.lvclass">)
        n128 = call <vilib>:"GetState.vi"("error in (no error)"=w363, "SMO"=w365) -> ("error out"=w361:errorcluster, "SMO State"=w360:T1, "SMO out"=w364:refnum<class "Instrument UI.lvclass">)  [unwired: 7 in]
        n129 = call <vilib>:"Clear Errors.vi"("error in (no error)"=w361) -> ("error out"=w362:errorcluster)  [unwired: 5 in, 1 out]
        n130 = case shown="\"Started\"" w360 {
          tunnel: [w371 w374] -> w366
          tunnel: w364 -> [_ w373]
          tunnel: w362 -> [w371 w372]
          frame Default {
          }
          frame "Started" {
            n131 = call <vilib>:"Show.vi"("error in (no error)"=w372, "SMO.UI"=w373) -> ("error out"=w374:errorcluster)  [unwired: 8 in, 1 out]
          }
        }
        n132 = call <vilib>:"Add State(s) to Queue__jki_lib_state_machine.vi"("State(s) in (\"\")"=w370) -> ("States Out"=w369:string)  [unwired: 14 in]
      }
      frame "SMO: Destroy Instrument" {
        # "Do not put any code in this frame.\n(It is a separator no-op. You can make a copy of this frame to create a new Macro frame)"
        n133 = Unbundle By Name(w382) -> ("Instrument"=w380:refnum<class "Instrument.lvclass">)
        n134 = call <vilib>:"GetState.vi"("error in (no error)"=w377, "SMO"=w380) -> ("error out"=w376:errorcluster, "SMO State"=w379:T1, "SMO out"=w375:refnum<class "Instrument.lvclass">)  [unwired: 7 in]
        n135 = call <vilib>:"Clear Errors.vi"("error in (no error)"=w376) -> ("error out"=w378:errorcluster)  [unwired: 5 in, 1 out]
        n136 = case shown="\"Stopped\"" w379 {
          tunnel: [w386 w389] -> w381
          tunnel: w378 -> [w386 w388]
          tunnel: w375 -> [_ w387]
          frame Default {
          }
          frame "Stopped" {
            n137 = call <vilib>:"Destroy.vi"("error in (no error)"=w388, "SMO"=w387) -> ("error out"=w389:errorcluster)  [unwired: 9 in]
          }
        }
        n138 = call <vilib>:"Add State(s) to Queue__jki_lib_state_machine.vi"("State(s) in (\"\")"=w385) -> ("States Out"=w384:string)  [unwired: 14 in]
      }
      frame "SMO: Hide Instrument UI" {
        # "Do not put any code in this frame.\n(It is a separator no-op. You can make a copy of this frame to create a new Macro frame)"
        n139 = Unbundle By Name(w397) -> ("Instrument UI"=w395:refnum<class "Instrument UI.lvclass">)
        n140 = call <vilib>:"GetState.vi"("error in (no error)"=w393, "SMO"=w395) -> ("error out"=w391:errorcluster, "SMO State"=w390:T1, "SMO out"=w394:refnum<class "Instrument UI.lvclass">)  [unwired: 7 in]
        n141 = call <vilib>:"Clear Errors.vi"("error in (no error)"=w391) -> ("error out"=w392:errorcluster)  [unwired: 5 in, 1 out]
        n142 = case shown="Default" w390 {
          tunnel: [w401 w404] -> w396
          tunnel: w394 -> [_ w403]
          tunnel: w392 -> [w401 w402]
          frame Default {
          }
          frame "Started" {
            n143 = call <vilib>:"Hide.vi"("error in (no error)"=w402, "SMO.UI"=w403) -> ("error out"=w404:errorcluster)  [unwired: 8 in, 1 out]
          }
        }
        n144 = call <vilib>:"Add State(s) to Queue__jki_lib_state_machine.vi"("State(s) in (\"\")"=w400) -> ("States Out"=w399:string)  [unwired: 14 in]
      }
      frame "SMO: Stop Instrument UI" {
        # "Do not put any code in this frame.\n(It is a separator no-op. You can make a copy of this frame to create a new Macro frame)"
        n145 = Unbundle By Name(w411) -> ("Instrument UI"=w406:refnum<class "Instrument UI.lvclass">)
        n146 = call <vilib>:"GetState.vi"("error in (no error)"=w410, "SMO"=w406) -> ("error out"=w409:errorcluster, "SMO State"=w407:T1, "SMO out"=w405:refnum<class "Instrument UI.lvclass">)  [unwired: 7 in]
        n147 = call <vilib>:"Clear Errors.vi"("error in (no error)"=w409) -> ("error out"=w408:errorcluster)  [unwired: 5 in, 1 out]
        n148 = case shown="\"Created\", \"Started\"" w407 {
          tunnel: [w416 w419] -> w412
          tunnel: w405 -> [_ w418]
          tunnel: w408 -> [w416 w417]
          frame Default {
          }
          frame "Created", "Started" {
            n149 = call <vilib>:"Stop.vi"("error in (no error)"=w417, "SMO"=w418) -> ("error out"=w419:errorcluster)  [unwired: 8 in, 1 out]
          }
        }
        n150 = call <vilib>:"Add State(s) to Queue__jki_lib_state_machine.vi"("State(s) in (\"\")"=w415) -> ("States Out"=w414:string)  [unwired: 14 in]
      }
      frame "SMO: Stop Instrument" {
        # "Do not put any code in this frame.\n(It is a separator no-op. You can make a copy of this frame to create a new Macro frame)"
        n151 = Unbundle By Name(w426) -> ("Instrument"=w421:refnum<class "Instrument.lvclass">)
        n152 = call <vilib>:"GetState.vi"("error in (no error)"=w425, "SMO"=w421) -> ("error out"=w424:errorcluster, "SMO State"=w422:T1, "SMO out"=w420:refnum<class "Instrument.lvclass">)  [unwired: 7 in]
        n153 = call <vilib>:"Clear Errors.vi"("error in (no error)"=w424) -> ("error out"=w423:errorcluster)  [unwired: 5 in, 1 out]
        n154 = case shown="\"Created\", \"Started\"" w422 {
          tunnel: [w431 w434] -> w427
          tunnel: w420 -> [_ w433]
          tunnel: w423 -> [w431 w432]
          frame Default {
          }
          frame "Created", "Started" {
            n155 = call <vilib>:"Stop.vi"("error in (no error)"=w432, "SMO"=w433) -> ("error out"=w434:errorcluster)  [unwired: 8 in, 1 out]
          }
        }
        n156 = call <vilib>:"Add State(s) to Queue__jki_lib_state_machine.vi"("State(s) in (\"\")"=w430) -> ("States Out"=w429:string)  [unwired: 14 in]
      }
      frame "SMO: Destroy Instrument UI" {
        # "Do not put any code in this frame.\n(It is a separator no-op. You can make a copy of this frame to create a new Macro frame)"
        n157 = Unbundle By Name(w441) -> ("Instrument UI"=w440:refnum<class "Instrument UI.lvclass">)
        n158 = call <vilib>:"GetState.vi"("error in (no error)"=w438, "SMO"=w440) -> ("error out"=w437:errorcluster, "SMO State"=w435:T1, "SMO out"=w439:refnum<class "Instrument UI.lvclass">)  [unwired: 7 in]
        n159 = call <vilib>:"Clear Errors.vi"("error in (no error)"=w437) -> ("error out"=w436:errorcluster)  [unwired: 5 in, 1 out]
        n160 = case shown="Default" w435 {
          tunnel: w436 -> [w446 w449]
          tunnel: [w446 w448] -> w442
          tunnel: w439 -> [_ w447]
          frame Default {
          }
          frame "Stopped" {
            n161 = call <vilib>:"Destroy.vi"("error in (no error)"=w449, "SMO"=w447) -> ("error out"=w448:errorcluster)  [unwired: 9 in]
          }
        }
        n162 = call <vilib>:"Add State(s) to Queue__jki_lib_state_machine.vi"("State(s) in (\"\")"=w445) -> ("States Out"=w444:string)  [unwired: 14 in]
      }
      frame "---------- Splash ----------" {
        # "Template Separator\n(You can make a copy of, or modify, this frame)"
        n163 = call <vilib>:"Add State(s) to Queue__jki_lib_state_machine.vi"("State(s) in (\"\")"=w454) -> ("States Out"=w453:string)  [unwired: 14 in]
      }
      frame "Splash: Set Status" {
        # "Your code here.\n(You can make a copy of, or modify, this frame)"
        n164 = property on="Splash Status" class="Str"(error in=w457, "Value"=w458) -> (error out=w456:errorcluster)  [unwired: 1 in, 1 out]
        n165 = call <vilib>:"Add State(s) to Queue__jki_lib_state_machine.vi"("State(s) in (\"\")"=w461) -> ("States Out"=w460:string)  [unwired: 14 in]
      }
      frame "Splash: 2" {
        # "Your code here.\n(You can make a copy of, or modify, this frame)"
        n166 = call <vilib>:"Add State(s) to Queue__jki_lib_state_machine.vi"("State(s) in (\"\")"=w466) -> ("States Out"=w465:string)  [unwired: 14 in]
      }
    }
  }
  "error out" <- w2
